vi "Message Log.vi"(11 "Message":string) -> ()   [LabVIEW 2013, in "Yokogawa.lvlib" / "YKPZ400 Message Queue.lvlib"]
uses:
  YKPZ400 Message Queue.lvlib
  <vilib>/Utility/file.llb/Write To Spreadsheet File (string).vi
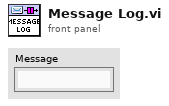
[diagram p1: front panel]
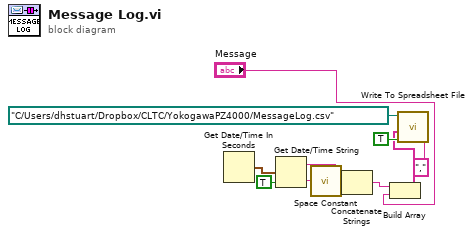
[diagram p0: block diagram]
diagram:
  n1 = Get Date/Time In Seconds() -> (seconds since 1Jan1904=w4:timestamp)
  n2 = Get Date/Time String(seconds (now)=w4, want seconds? (F)=TRUE) -> (date string=w6:string, time string=w7:string)  [unwired: 1 in]
  n3 = call <vilib>:"Space Constant.vi"() -> ("String"=w5:string)
  n4 = Concatenate Strings(w6, w5, w7) -> (w8:string)
  n5 = Build Array(w8, "Message") -> (w10:string[])
  n6 = call-poly <vilib>:"Write To Spreadsheet File.vi"("delimiter (\\t)"="," ("delimiter (\\t)"), "append to file? (new file:F)"=TRUE, "1D data"=w10, "file path (dialog if empty)"=path "C:/Users/dhstuart/Dropbox/CLTC/YokogawaPZ4000/MessageLog.csv") -> ()  [unwired: 4 in, 1 out]
